vi "Measure.vi"(8 "error in (no error)":errorcluster, 9 "measurement configuration":variant, 10 "measure call context in":refnum<class "Measure Call Context.lvclass">, 11 "measurement plugin in":refnum<class "WorkflowDO.lvclass">) -> (0 "error out":errorcluster, 1 "measurement results":variant, 2 "measure call context out":refnum<class "Measure Call Context.lvclass">, 3 "measurement plugin out":refnum<class "WorkflowDO.lvclass">)   [LabVIEW 2025, in "WorkflowDO.lvclass"]
uses:
  WorkflowDO.lvclass
  <vilib>/Plug-In SDKs/Measurements/Measure Call Context/Measure Call Context.lvclass
  Measurement Configuration.ctl
  WorkflowDO.lvclass/WorkflowDO.ctl
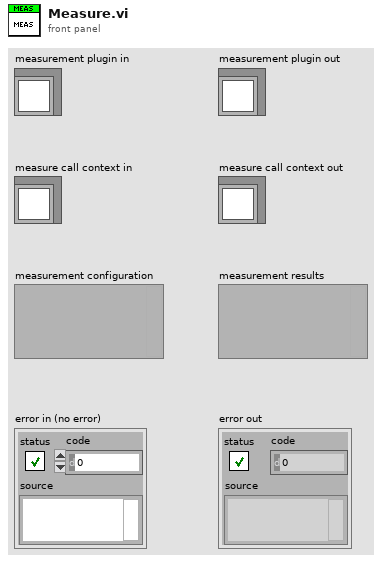
[diagram p1: front panel]
types:
  T1 = typedef "WorkflowDO.lvclass/Measurement Configuration.ctl" = cluster{"Counter Resource Name":string, "Output Resource Name":string, "Frequency":dbl, "Duty Cycle":dbl, "Number of Pulses":i32}
  T2 = typedef "WorkflowDO.lvclass/Measurement Results.ctl" = cluster{"Actual Frequency":dbl, "Actual Duty Cycle":dbl}
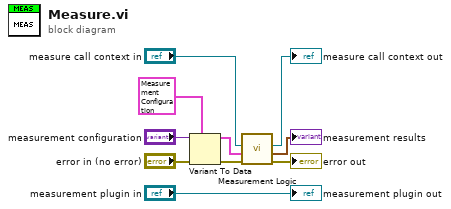
[diagram p0: block diagram]
diagram:
  n1 = Variant To Data(error in="error in (no error)", type=T1 {"Counter Resource Name"="Lorem ipsum dolor sit", "Output Resource Name"="/Dev1/PFI12", "Frequency"=1.2, "Duty Cycle"=32.0, "Number of Pulses"=64} ("measurement configuration"), Variant="measurement configuration") -> (data=w1:T1, error out=w7:errorcluster)
  n2 = call "Measurement Logic.vi"("error in"=w7, "measurement configuration"=w1, "measure call context in"="measure call context in") -> ("error out"=→"error out":errorcluster, "measurement results"=→"measurement results":T2, "measure call context out"=→"measure call context out":refnum<class "Measure Call Context.lvclass">)  [unwired: 6 in]
  "measurement plugin out" <- "measurement plugin in"
